vi "display queue to fp display_MD.vi"() -> ()   [LabVIEW 2012]
uses:
  <vilib>/Utility/VariantDataType/Type.ctl
  GFG/GFGnumericGet.vi
  GFG/GFGImageRefsGet.vi
  GFG/GFGDisplayRefsGet.vi
  GFG/GFGbooleanGet.vi
  GFG/GFG library.lvlib
  <vilib>/Utility/VariantDataType/VariantType.lvlib
panel:
  out "error out 2":errorcluster
  out "size(s)":i32[](array[numeric])
  out "# elements in display data queue":i32
  out "error out":errorcluster
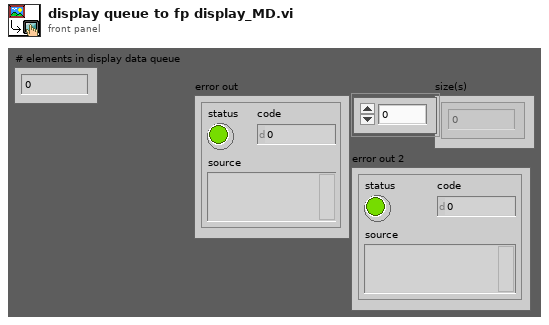
[diagram p1: front panel]
types:
  T1 = cluster{"NewVal":bool, "Event Registration Refnum":refnum<event-registration>}
  T2 = cluster{"Channel 1 small":refnum<vi>, "Channel 2 small":refnum<vi>, "Channel 3 small":refnum<vi>, "Channel 4 small":refnum<vi>, "Channel 1 large":refnum<vi>, "Channel 2 large":refnum<vi>, "Channel 3 large":refnum<vi>, "Channel 4 large":refnum<vi>, "RGB overlay":refnum<vi>, "ROI Image display":refnum<vi>, "arb line scan display":refnum<vi>, "Channel 5 large":refnum<vi>}
  T3 = typedef "IMAQ Image.ctl" = refnum<image>
  T4 = cluster{"Channel 1 small":T3, "Channel 2 small":T3, "Channel 3 small":T3, "Channel 4 small":T3, "Channel 1 large":T3, "Channel 2 large":T3, "Channel 3 large":T3, "Channel 4 large":T3, "RGB overlay":T3, "ROI Image display":T3, "arb line scan display":T3, "Channel 5 large":T3}
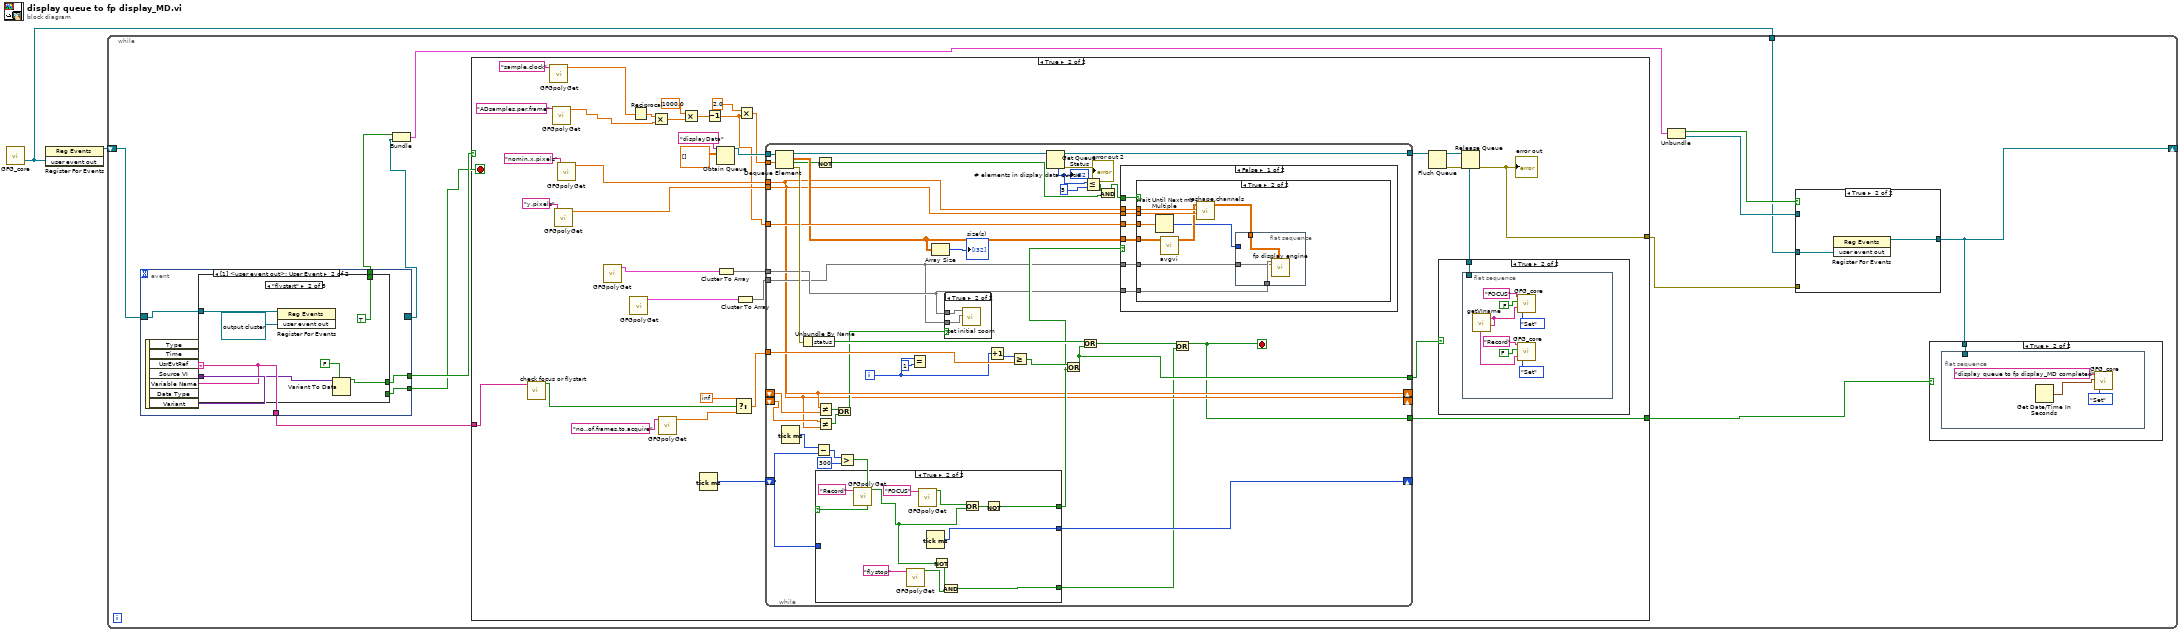
[diagram p0: block diagram]
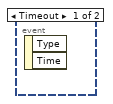
[diagram p4: hidden frame]
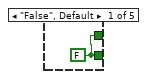
[diagram p5: hidden frame]
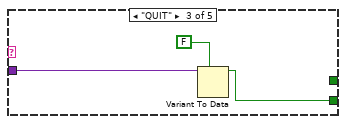
[diagram p6: hidden frame]
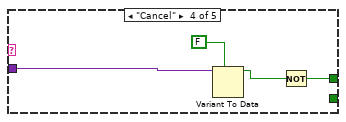
[diagram p7: hidden frame]
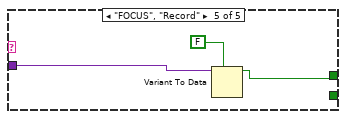
[diagram p8: hidden frame]
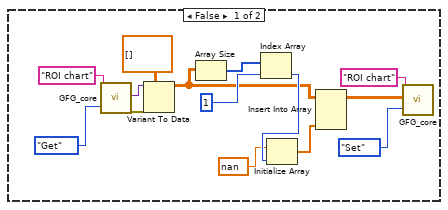
[diagram p12: hidden frame]
diagram:
  n1 = call "GFG_core.vi"() -> ("user event out"=w1:refnum<user-event>)  [unwired: 13 in, 6 out]
  n2 = register-events(w1) -> (reference out=w2:refnum<event-registration>)  [unwired: 2 in, 1 out]
  n3 = while {
    shift-right: [w4] -> _
    shift-left: w2 -> [w15]
    tunnel: w1 -> [w6]
    stop <- w13 stop-if-true
    n4 = event shown="[1] <user event out>: User Event" {
      selector: w15 -> [_ w24]
      dyn-events: [_ _] -> w11
      timeout: _ -> [_ _]
      tunnel: [_ w28] -> w14
      tunnel: [_ w27] -> w13
      tunnel: [_ w25] -> w5
      tunnel: [_ w23] -> w12
      event Timeout {
        n5 = event-data() -> ()  [unwired: 1 in, 2 out]
      }
      event User Event {
        n6 = event-data() -> ("Variable Name"=w25:string, "Variant"=w26:variant)  [unwired: 1 in, 5 out]
        n7 = case shown="\"flystart\"" w25 {
          tunnel: [w29 w33 _ w39 w43] -> w28
          tunnel: [w29 _ w36 _ _] -> w27
          tunnel: w26 -> [_ w34 w38 w41 w44]
          tunnel: w24 -> [_ w31 _ _ _]
          tunnel: [_ TRUE ("NewVal") _ _ _] -> w23
          frame "False", Default {
            w29 = FALSE ("NewVal")
          }
          frame "flystart" {
            n8 = register-events(reference=w31, refnum<user-event> refnum ("user event out")) -> ()  [unwired: 1 in, 2 out]
            n9 = Variant To Data(type=FALSE ("NewVal"), Variant=w34) -> (data=w33:bool)  [unwired: 1 in, 1 out]
          }
          frame "QUIT" {
            n10 = Variant To Data(type=FALSE ("NewVal"), Variant=w38) -> (data=w36:bool)  [unwired: 1 in, 1 out]
          }
          frame "Cancel" {
            n11 = Variant To Data(type=FALSE ("NewVal"), Variant=w41) -> (data=w40:bool)  [unwired: 1 in, 1 out]
            n12 = Not(x=w40) -> (.not. x?=w39:bool)
          }
          frame "FOCUS", "Record" {
            n13 = Variant To Data(type=FALSE ("NewVal"), Variant=w44) -> (data=w43:bool)  [unwired: 1 in, 1 out]
          }
        }
      }
    }
    n14 = Bundle("NewVal"=w12, "Event Registration Refnum"=w11) -> (w9:T1)  [unwired: 1 in]
    n15 = case shown="True" w14 {
      tunnel: [_ w54] -> w10
      tunnel: w5 -> [_ w49]
      tunnel: [_ w46] -> w3
      frame False {
      }
      frame True {
        n16 = call "check focus or flystart.vi"("x"=w49) -> ("x .or. y?"=w48:bool)  [unwired: 10 in]
        n17 = call-poly "GFGpolyGet.vi"("Variable Name in"="sample.clock" ("Tag in")) -> ("Numeric"=w72:dbl)  [unwired: 9 in, 1 out]
        n18 = call-poly "GFGpolyGet.vi"("Variable Name in"="ADsamples.per.frame" ("Tag in")) -> ("Numeric"=w56:dbl)  [unwired: 9 in, 1 out]
        n19 = call-poly "GFGpolyGet.vi"("Variable Name in"="y.pixels") -> ("Numeric"=w58:dbl)  [unwired: 9 in, 1 out]
        n20 = call-poly "GFGpolyGet.vi"("Variable Name in"="nomin.x.pixels") -> ("Numeric"=w59:dbl)  [unwired: 9 in, 1 out]
        n21 = call-poly "GFGpolyGet.vi"() -> ("DisplayRefsOut(generic class)"=w68:T2)  [unwired: 10 in, 1 out]
        n22 = call-poly "GFGpolyGet.vi"() -> ("Image Refs Out"=w67:T4)  [unwired: 10 in, 1 out]
        n23 = Reciprocal(x=w72) -> (1/x=w77:dbl)
        n24 = Multiply(x=w77, y=w56) -> (x*y=w76:dbl)
        n25 = call-poly "GFGpolyGet.vi"("Variable Name in"="no..of.frames.to.acquire" ("Tag in")) -> ("Numeric"=w51:dbl)  [unwired: 9 in, 1 out]
        n26 = Multiply(x=1000.0, y=w76) -> (x*y=w74:dbl)
        n27 = Tick Count (ms)() -> (millisecond timer value=w57:u32)
        n28 = Decrement(x=w74) -> (x-1=w55:dbl)
        n29 = Obtain Queue(name (unnamed)="displayData", element data type=dbl[][] [] ("y backward image")) -> (queue out=w69:refnum<queue>)  [unwired: 3 in, 2 out]
        n30 = Cluster To Array(cluster=w68) -> (array=w65:refnum<vi>[])
        n31 = Select(t=inf, s=w48, f=w51) -> (s? t:f=w50:dbl)
        n32 = Cluster To Array(cluster=w67) -> (array=w66:T3[])
        n33 = Multiply(x=2.0, y=w55) -> (x*y=w64:dbl)
        n34 = while {
          tunnel: [w122] -> w62
          tunnel: w50 -> [w128]
          tunnel: w64 -> [w124]
          tunnel: w69 -> [w125]
          tunnel: w65 -> [w111]
          tunnel: w66 -> [w101]
          tunnel: w59 -> [w93]
          tunnel: w58 -> [w99]
          shift-right: [w116] -> _
          shift-left: w57 -> [w115]
          tunnel: w55 -> [w110]
          tunnel: [w91] -> w47
          shift-right: [w99] -> _
          shift-left: _ -> [w98]
          shift-right: [w93] -> _
          shift-left: _ -> [w96]
          tunnel: [w90] -> w46
          i -> [w113]
          stop <- w90 stop-if-true
          n35 = Dequeue Element(queue=w125, timeout in ms (-1)=w124) -> (queue out=w123:refnum<queue>, element=w106:dbl[][], timed out?=w103:bool, error out=w127:errorcluster)  [unwired: 1 in]
          n36 = Tick Count (ms)() -> (millisecond timer value=w120:u32)
          n37 = Unbundle By Name(w127) -> ("status"=w129:bool)
          n38 = Subtract(x=w120, y=w115) -> (x-y=w119:u32)
          n39 = Not(x=w103) -> (.not. x?=w102:bool)
          n40 = Not Equal?(x=w99, y=w98) -> (x != y?=w97:bool)
          n41 = Not Equal?(x=w96, y=w93) -> (x != y?=w94:bool)
          n42 = Or(x=w97, y=w94) -> (x .or. y?=w95:bool)
          n43 = Greater?(x=w119, y=u32 300) -> (0:w117:bool)
          n44 = case shown="True" w117 {
            tunnel: [_ w166] -> w114
            tunnel: [w165 w172] -> w116
            tunnel: w115 -> [w165 _]
            tunnel: [_ w167] -> w89
            frame False {
            }
            frame True {
              n45 = call-poly "GFGpolyGet.vi"("Variable Name in"="Record") -> ("Boolean"=w168:bool)  [unwired: 10 in]
              n46 = call-poly "GFGpolyGet.vi"("Variable Name in"="flystop") -> ("Boolean"=w169:bool)  [unwired: 10 in]
              n47 = call-poly "GFGpolyGet.vi"("Variable Name in"="FOCUS") -> ("Boolean"=w175:bool)  [unwired: 10 in]
              n48 = Tick Count (ms)() -> (millisecond timer value=w172:u32)
              n49 = Not(x=w168) -> (.not. x?=w170:bool)
              n50 = And(x=w170, y=w169) -> (x .and. y?=w167:bool)
              n51 = Or(x=w175, y=w168) -> (x .or. y?=w176:bool)
              n52 = Not(x=w176) -> (.not. x?=w166:bool)
            }
          }
          n53 = Equal?(x=w113, y=1) -> ()  [unwired: 1 out]
          n54 = Array Size(array=w106) -> (size(s)=→"size(s)":i32[])
          n55 = case shown="True" w95 {
            tunnel: w111 -> [_ w131]
            tunnel: w101 -> [_ w130]
            frame False {
            }
            frame True {
              n56 = call "set initial zoom.vi"("Image Refs In"=w130, "DisplayRefsIn(generic class)"=w131) -> ()  [unwired: 10 in]
            }
          }
          n57 = Increment(x=w113) -> (x+1=w121:i32)
          n58 = Greater Or Equal?(x=w121, y=w128) -> (x >= y?=w126:bool)
          n59 = Get Queue Status(queue=w123) -> (queue out=w122:refnum<queue>, error out=→"error out 2":errorcluster, # elements in queue=w109:i32)  [unwired: 2 in, 5 out]
          "# elements in display data queue" <- w109
          n60 = Or(x=w126, y=w114) -> (x .or. y?=w91:bool)
          n61 = Or(x=w129, y=w91) -> (x .or. y?=w92:bool)
          n62 = Less Or Equal?(x=w109, y=5) -> (x <= y?=w107:bool)
          n63 = And(x=w107, y=w102) -> (x .and. y?=w104:bool)
          n64 = case shown="False" w114 {
            tunnel: w93 -> [w138 _]
            tunnel: w99 -> [w137 _]
            tunnel: w106 -> [w136 _]
            tunnel: w111 -> [w135 _]
            tunnel: w101 -> [w134 _]
            tunnel: w110 -> [w133 _]
            tunnel: w104 -> [w132 _]
            frame False {
              n65 = case shown="True" w132 {
                tunnel: w138 -> [_ w161]
                tunnel: w137 -> [_ w160]
                tunnel: w136 -> [_ w159]
                tunnel: w135 -> [_ w156]
                tunnel: w134 -> [_ w155]
                tunnel: w133 -> [_ w154]
                frame False {
                  n66 = call "GFG_core.vi"("Variable Name in"="ROI chart", "Action"=enum16{"Init", "Set", "Get"}."Get") -> ("Variant Out"=w149:variant, "error out"=w150:errorcluster)  [unwired: 11 in, 5 out]
                  n67 = Variant To Data(error in=w150, type=sgl[][] [] ("y backward image"), Variant=w149) -> (data=w144:sgl[][])  [unwired: 1 out]
                  n68 = Array Size(array=w144) -> (size(s)=w142:i32[])
                  n69 = Index Array(array=w142, index=1) -> (element=w146:i32)
                  n70 = Initialize Array(nan, w146) -> (w143:dbl[])
                  n71 = Insert Into Array(array=w144, new element=w143) -> (w139:sgl[][])  [unwired: 2 in]
                  n72 = call "GFG_core.vi"("Variable Name in"="ROI chart", "Variant in"=w139, "Action"=enum16{"Init", "Set", "Get"}."Set") -> ()  [unwired: 10 in, 7 out]
                }
                frame True {
                  n73 = Wait Until Next ms Multiple(millisecond multiple=w154) -> (millisecond timer value=w153:u32)
                  n74 = call "avgvi.vi"("image in"=w159) -> ("image out"=w158:sgl[][])  [unwired: 10 in]
                  n75 = call "reshape.channels.vi"("y.pixels"=w160, "x.pixels"=w161, "element"=w158) -> ("Array"=w157:dbl[][][])  [unwired: 8 in]
                  n76 = flat-sequence {
                    tunnel: w157 -> [w164]
                    tunnel: w156 -> [w163]
                    tunnel: w155 -> [w162]
                    tunnel: w153 -> [_]
                    frame #0 {
                      n77 = call "fp display engine.vi"("channel data in"=w164, "Image Refs In"=w162, "DisplayRefsIn(generic class)"=w163) -> ()  [unwired: 9 in]
                    }
                  }
                }
              }
            }
            frame True {
            }
          }
          n78 = Or(x=w92, y=w89) -> (x .or. y?=w90:bool)
        }
        n79 = Flush Queue(queue=w62) -> (queue out=w80:refnum<queue>, error out=w79:errorcluster)  [unwired: 1 in, 1 out]
        n80 = case shown="True" w47 {
          tunnel: w62 -> [_ w81]
          frame False {
          }
          frame True {
            n81 = flat-sequence {
              tunnel: w81 -> [_]
              frame #0 {
                n82 = call "getVIname.vi"() -> ("VI name"=w82:string)  [unwired: 19 in]
                n83 = call "GFG_core.vi"("Variable Name in"="Record" ("Tag in"), "Variant in"=FALSE, "Source VI"=w82, "Action"=enum16{"Init", "Set", "Get"}."Set") -> ()  [unwired: 9 in, 7 out]
                n84 = call "GFG_core.vi"("Variable Name in"="FOCUS" ("Tag in"), "Variant in"=FALSE, "Source VI"=w82, "Action"=enum16{"Init", "Set", "Get"}."Set") -> ()  [unwired: 9 in, 7 out]
              }
            }
          }
        }
        n85 = Release Queue(queue=w80, error in (no error)=w79) -> (error out=w54:errorcluster)  [unwired: 1 in, 2 out]
        "error out" <- w54
      }
    }
    n86 = Unbundle(w9) -> ("NewVal"=w8:bool, "Event Registration Refnum"=w7:refnum<event-registration>)
    n87 = case shown="True" w8 {
      tunnel: [w20 w22] -> w4
      tunnel: w6 -> [_ w21]
      tunnel: w10 -> [_ _]
      tunnel: w7 -> [w20 _]
      frame False {
      }
      frame True {
        n88 = register-events(w21) -> (reference out=w22:refnum<event-registration>)  [unwired: 2 in, 1 out]
      }
    }
    n89 = case shown="True" w3 {
      tunnel: w4 -> [_ w16]
      frame False {
      }
      frame True {
        n90 = flat-sequence {
          tunnel: w16 -> [_]
          frame #0 {
            n91 = Get Date/Time In Seconds() -> (seconds since 1Jan1904=w17:timestamp)
            n92 = call "GFG_core.vi"("Variable Name in"="display queue to fp display_MD completed", "Variant in"=w17, "Action"=enum16{"Init", "Set", "Get"}."Set") -> ()  [unwired: 10 in, 7 out]
          }
        }
      }
    }
  }
